vi "ToggleByRoomName.vi"(0 "reference in":refnum<class "LightingSystem.lvclass">, 2 "RoomName":string, 5 "Error In":errorcluster) -> (14 "reference out":refnum<class "LightingSystem.lvclass">, 19 "Error Out":errorcluster)   [LabVIEW 2024, in "LightingSystem.lvclass"]
doc: "Takes RoomName string parameter and toggle elements of that room"
uses:
  LightingSystem.lvclass
  House/Room_class/Room.lvclass
  Devices/Light_class/Light.lvclass
panel:
  # "Connector Pane"
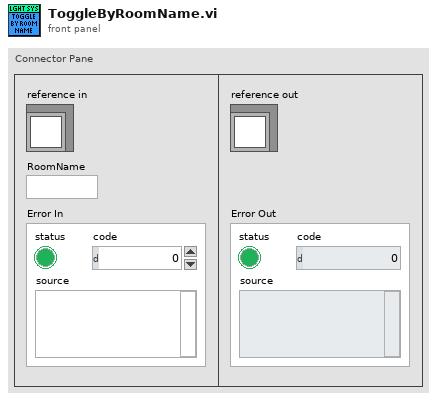
[diagram p1: front panel]
types:
  T1 = typedef "LightingSystem.lvclass/ObjectAttributes.ctl" = cluster{"Rooms":T2}
  T2 = typedef "Rooms Map.ctl" = map{string, refnum<class "Room.lvclass">}
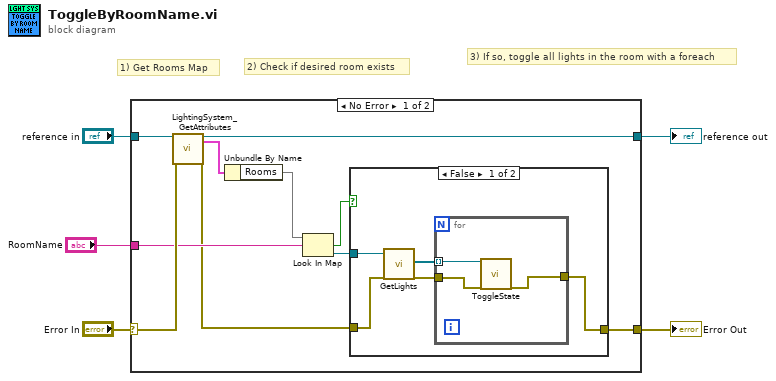
[diagram p0: block diagram]
diagram:
  # "3) If so, toggle all lights in the room with a foreach"
  # "2) Check if desired room exists"
  # "1) Get Rooms Map"
  n1 = case shown="No Error" "Error In" {
    selector: "Error In" -> [w14 w26]
    tunnel: [w7 w26] -> w4
    tunnel: [w13 w25] -> w2
    tunnel: "reference in" -> [w15 w25]
    tunnel: "RoomName" -> [w12 _]
    frame No Error {
      n2 = call "LightingSystem_GetAttributes.vi"("reference in"=w15, "Error In"=w14) -> ("reference out"=w13:refnum<class "LightingSystem.lvclass">, "Data"=w8:T1, "Error Out"=w6:errorcluster)  [unwired: 14 in, 1 out]
      n3 = Unbundle By Name(w8) -> ("Rooms"=w11:T2)
      n4 = Look In Map(map=w11, key=w12) -> (key not found?=w10:bool, value=w9:refnum<class "Room.lvclass">)  [unwired: 1 in]
      n5 = case shown="False" w10 {
        tunnel: w9 -> [w20 _]
        tunnel: w6 -> [w17 w24]
        tunnel: [w16 w24] -> w7
        frame False {
          n6 = call-dynamic "GetLights.vi"("reference in"=w20, "Error In"=w17) -> ("Lights"=w19:refnum<class "Light.lvclass">[], "Error Out"=w18:errorcluster)  [unwired: 15 in, 1 out]
          n7 = for {
            tunnel: w19 -> [w23] mode=indexing
            tunnel: w18 -> [w22]
            tunnel: [w21] -> w16
            n8 = call "ToggleState.vi"("reference in"=w23, "Error In"=w22) -> ("Error Out"=w21:errorcluster)  [unwired: 16 in, 1 out]
          }
        }
        frame True {
        }
      }
    }
    frame Error {
    }
  }
  "Error Out" <- w4
  "reference out" <- w2
